vi "Find CAN_ID.vi"(8 "error in (no error)":errorcluster, 11 "A2L Text In":string[](array[string])) -> (0 "error out":errorcluster, 2 "DTO_ID":u32[](array[numeric]))   [LabVIEW 2019, in "A2L Utility.lvlib"]
uses:
  A2L Utility.lvlib
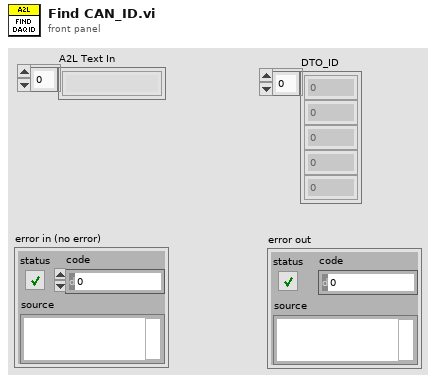
[diagram p1: front panel]
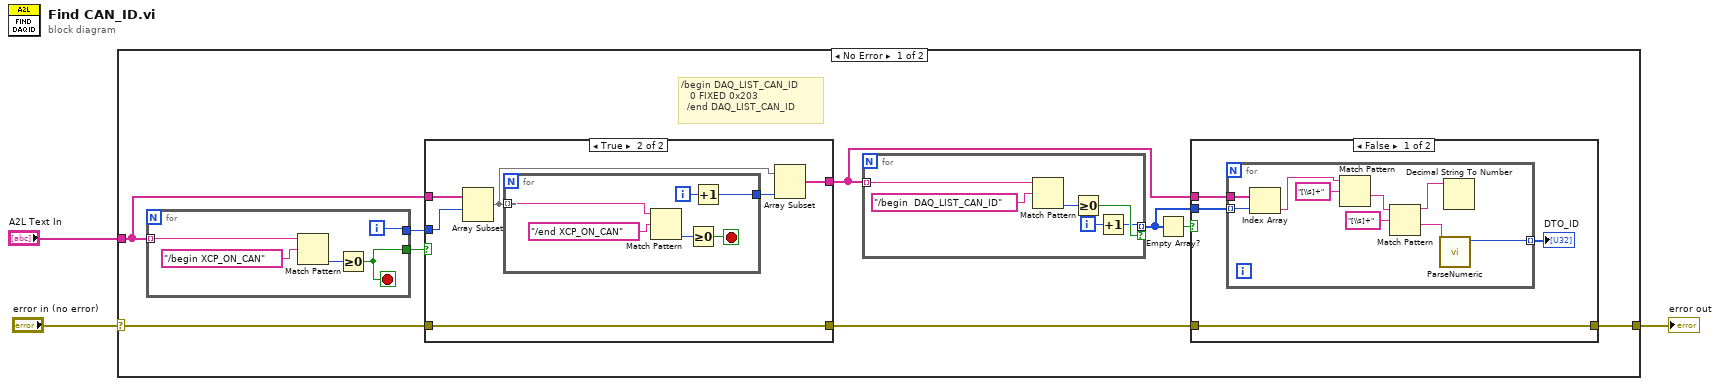
[diagram p0: block diagram]
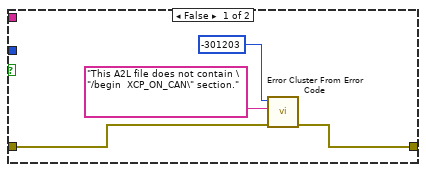
[diagram p2: hidden frame]
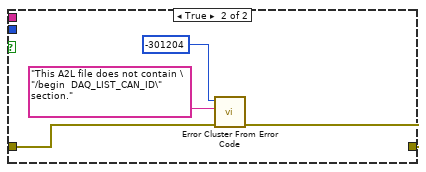
[diagram p3: hidden frame]
diagram:
  n1 = case shown="No Error" "error in (no error)" {
    selector: "error in (no error)" -> [w9 w57]
    tunnel: "A2L Text In" -> [w12 _]
    tunnel: [w4 w57] -> w2
    frame No Error {
      # "/begin DAQ_LIST_CAN_ID\n\t\t\t0 FIXED 0x203\n\t\t/end DAQ_LIST_CAN_ID"
      n2 = for {
        tunnel: w12 -> [w33] mode=indexing
        tunnel: [w31] -> w11
        tunnel: [w29] -> w10
        i -> [w29]
        stop <- w31 stop-if-true
        n3 = Match Pattern(string=w33, regular expression="/begin XCP_ON_CAN") -> (offset past match=w30:i32)  [unwired: 1 in, 3 out]
        n4 = Greater Or Equal To 0?(x=w30) -> (x >= 0?=w31:bool)
      }
      n5 = case shown="True" w11 {
        tunnel: w12 -> [_ w22]
        tunnel: w10 -> [_ w21]
        tunnel: w9 -> [w16 w18]
        tunnel: [w15 w18] -> w8
        tunnel: [_ w19] -> w6
        frame False {
          n6 = call <vilib>:"Error Cluster From Error Code.vi"("error in (no error)"=w16, "error message (\"\")"="This A2L file does not contain \"/begin  XCP_ON_CAN\" section." ("error message (\"\")"), "error code (0)"=-301203) -> ("error out"=w15:errorcluster)  [unwired: 6 in]
        }
        frame True {
          n7 = Array Subset(array=w22, index=w21) -> (w17:string[])  [unwired: 1 in]
          n8 = for {
            tunnel: w17 -> [w23] mode=indexing
            tunnel: [w25] -> w20
            i -> [w26]
            stop <- w24 stop-if-true
            n9 = Match Pattern(string=w23, regular expression="/end XCP_ON_CAN") -> (offset past match=w27:i32)  [unwired: 1 in, 3 out]
            n10 = Greater Or Equal To 0?(x=w27) -> (x >= 0?=w24:bool)
            n11 = Increment(x=w26) -> (x+1=w25:i32)
          }
          n12 = Array Subset(array=w17, length=w20) -> (w19:string[])  [unwired: 1 in]
        }
      }
      n13 = for {
        tunnel: w6 -> [w39] mode=indexing
        tunnel: [w34] -> w5 mode=indexing if=w35
        i -> [w36]
        n14 = Match Pattern(string=w39, regular expression="/begin  DAQ_LIST_CAN_ID") -> (offset past match=w37:i32)  [unwired: 1 in, 3 out]
        n15 = Greater Or Equal To 0?(x=w37) -> (x >= 0?=w35:bool)
        n16 = Increment(x=w36) -> (x+1=w34:i32)
      }
      n17 = Empty Array?(array=w5) -> (empty?=w7:bool)
      n18 = case shown="False" w7 {
        tunnel: w6 -> [w43 _]
        tunnel: w8 -> [w42 w56]
        tunnel: [w42 w55] -> w4
        tunnel: w5 -> [w41 _]
        frame False {
          n19 = for {
            tunnel: w43 -> [w52]
            tunnel: w41 -> [w51] mode=indexing
            tunnel: [w44] -> w40 mode=indexing
            n20 = Index Array(array=w52, index=w51) -> (element=w50:string)
            n21 = Match Pattern(string=w50, regular expression="[\\s]+") -> (after substring=w47:string)  [unwired: 1 in, 3 out]
            n22 = Match Pattern(string=w47, regular expression="[\\s]+") -> (before substring=w46:string, after substring=w45:string)  [unwired: 1 in, 2 out]
            n23 = call "ParseNumeric.vi"("String In"=w45) -> ("Numeric"=w44:u32)  [unwired: 10 in]
            n24 = Decimal String To Number(string=w46) -> ()  [unwired: 2 in, 2 out]
          }
          "DTO_ID" <- w40
        }
        frame True {
          n25 = call <vilib>:"Error Cluster From Error Code.vi"("error in (no error)"=w56, "error message (\"\")"="This A2L file does not contain \"/begin  DAQ_LIST_CAN_ID\" section." ("error message (\"\")"), "error code (0)"=-301204) -> ("error out"=w55:errorcluster)  [unwired: 6 in]
        }
      }
    }
    frame Error {
    }
  }
  "error out" <- w2
